vi "nelder_get_center_of_simplex.vi"(11 "simplex input":sgl[][](array[numeric])) -> (0 "area":sgl, 1 "min":sgl, 2 "z":sgl, 3 "y":sgl)   [LabVIEW 2018]
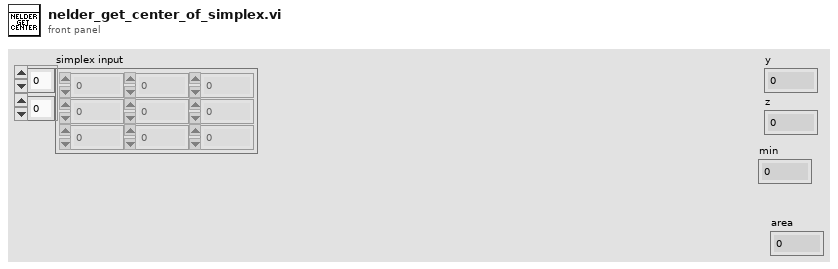
[diagram p1: front panel]
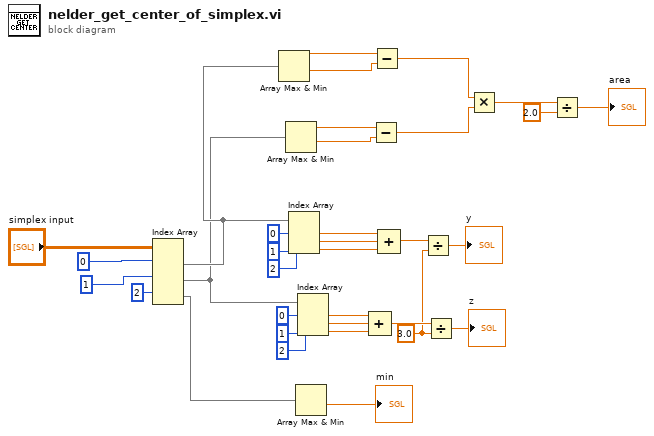
[diagram p0: block diagram]
diagram:
  w23 = sgl 3.0 ("y")
  n1 = Index Array(array="simplex input", index (row) #1=0 ("index (row)"), index (row) #2=1 ("index (row)"), index (row) #3=2 ("index (row)")) -> (element #1=w11:sgl[], element #2=w10:sgl[], element #3=w21:sgl[])  [unwired: 3 in]
  n2 = Array Max & Min(array=w11) -> (max value=w7:sgl, min value=w6:sgl)  [unwired: 2 out]
  n3 = Array Max & Min(array=w10) -> (max value=w9:sgl, min value=w8:sgl)  [unwired: 2 out]
  n4 = Index Array(array=w11, index #1=0 ("index"), index #2=1 ("index"), index #3=2 ("index")) -> (element #1=w16:sgl, element #2=w18:sgl, element #3=w19:sgl)
  n5 = Array Max & Min(array=w21) -> (min value=→"min":sgl)  [unwired: 3 out]
  n6 = Index Array(array=w10, index #1=0 ("index"), index #2=1 ("index"), index #3=2 ("index")) -> (element #1=w12:sgl, element #2=w13:sgl, element #3=w14:sgl)
  n7 = Compound Arithmetic op=ADD(w12, w13, w14) -> (w24:sgl)
  n8 = Subtract(x=w9, y=w8) -> (x-y=w5:sgl)
  n9 = Subtract(x=w7, y=w6) -> (x-y=w4:sgl)
  n10 = Compound Arithmetic op=ADD(w16, w18, w19) -> (w25:sgl)
  n11 = Divide(x=w25, y=w23) -> (x/y=→"y":sgl)
  n12 = Divide(x=w24, y=w23) -> (x/y=→"z":sgl)
  n13 = Multiply(x=w4, y=w5) -> (x*y=w3:sgl)
  n14 = Divide(x=w3, y=sgl 2.0) -> (x/y=→"area":sgl)
